vi "Open Current VI Location.vi"(6 "Variant in":variant, 7 "Shift Pressed?":bool, 8 "error in (no error)":errorcluster, 10 "QD Combo Box Ref":refnum<vi>, 11 "QD Launch VI Ref":refnum<vi>) -> (0 "error out":errorcluster, 4 "Variant out":variant)   [LabVIEW 2017, in "Smart Open VI Location.lvlib"]
doc: "Open Current VI Location in Explorer Window."
uses:
  Smart Open VI Location.lvlib
panel:
  in  "Undo Name":string="NEVSTOP__OpenFileLocaiton"
  # "Do not change the connector pane of this VI.\n\nSee the block diagram for directions on how to use this template."
  # "Specify the name of the Undo transaction"
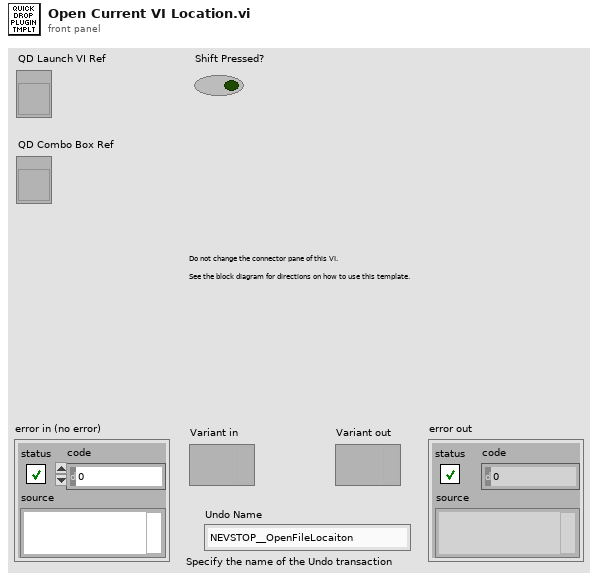
[diagram p1: front panel]
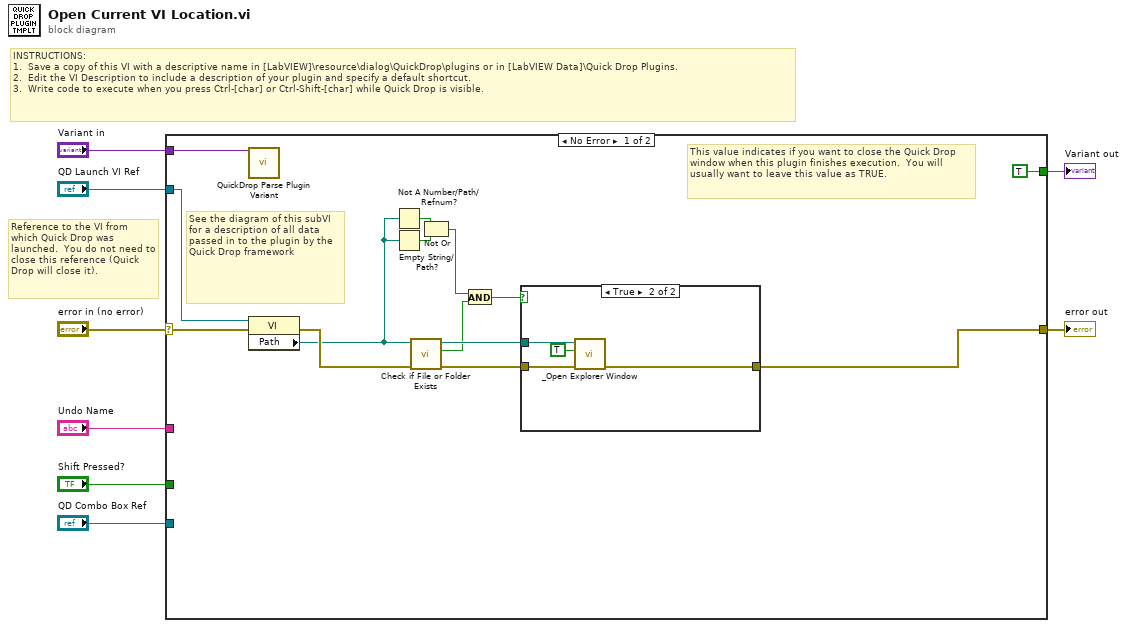
[diagram p0: block diagram]
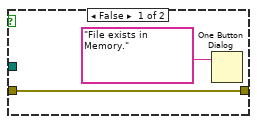
[diagram p2: hidden frame]
diagram:
  # "Reference to the VI from which Quick Drop was launched.  You do not need to close this reference (Quick Drop will close it)."
  # "INSTRUCTIONS:\n1.  Save a copy of this VI with a descriptive name in [LabVIEW]\\resource\\dialog\\QuickDrop\\plugins or in [LabVIEW Data]\\Quick Drop Plugins.\n2.  Edit the VI Description to include a description of your plugin and specify a default shortcut. \n3.  Write code to execute when you press Ctrl-[char] or Ctrl-Shift-[char] while Quick Drop is visible."
  n1 = case shown="No Error" "error in (no error)" {
    selector: "error in (no error)" -> [w21 w29]
    tunnel: [w18 w29] -> w7
    tunnel: "QD Launch VI Ref" -> [w20 _]
    tunnel: "Shift Pressed?" -> [_ _]
    tunnel: "QD Combo Box Ref" -> [_ _]
    tunnel: "Variant in" -> [w22 _]
    tunnel: "Undo Name" -> [_ _]
    tunnel: [TRUE _] -> w1
    frame No Error {
      # "This value indicates if you want to close the Quick Drop window when this plugin finishes execution.  You will usually want to leave this value as TRUE."
      # "See the diagram of this subVI for a description of all data passed in to the plugin by the Quick Drop framework"
      n2 = call <vilib>:"QuickDrop Parse Plugin Variant.vi"("QDKS Variant in"=w22) -> ()  [unwired: 12 in, 3 out]
      n3 = property class="VI"(reference=w20, error in=w21) -> (error out=w16:errorcluster, "Path"=w12:path)  [unwired: 1 out]
      n4 = Not A Number/Path/Refnum?(number/path/refnum=w12) -> (NaN/Path/Refnum?=w10:bool)
      n5 = Empty String/Path?(string/path=w12) -> (empty?=w9:bool)
      n6 = call <vilib>:"Check if File or Folder Exists.vi"("error in (no error)"=w16, "path"=w12) -> ("error out"=w15:errorcluster, "file or folder exists?"=w13:bool, "dup path"=w17:path)  [unwired: 7 in]
      n7 = Not Or(1:w9, 2:w10) -> (0:w14:bool)
      n8 = And(x=w14, y=w13) -> (x .and. y?=w11:bool)
      n9 = case shown="True" w11 {
        tunnel: [w24 w27] -> w18
        tunnel: w17 -> [_ w26]
        tunnel: w15 -> [w24 w25]
        frame False {
          n10 = One Button Dialog(message="File exists in Memory.") -> ()  [unwired: 1 in, 1 out]
        }
        frame True {
          n11 = call "_Open Explorer Window.vi"("error in (no error)"=w25, "Select Directory? (F: Open Directory)"=TRUE, "Directory or File"=w26) -> ("error out"=w27:errorcluster)  [unwired: 8 in]
        }
      }
    }
    frame Error {
    }
  }
  "error out" <- w7
  "Variant out" <- w1
